vi "UpdateGraphsTableDisplay.vi"(9 "MainMenu_In":refnum<vi>, 10 "DisplayGraphsTable_In":refnum<vi>, 11 "Output Values of Device":refnum<vi>) -> ()   [LabVIEW 2013]
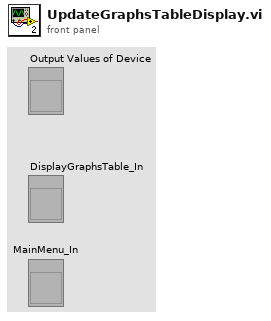
[diagram p1: front panel]
types:
  T1 = typedef "DysplayGraph.ctl" = cluster{"Graph":cluster{"X":dbl, "Y":dbl}[], "X is":u16, "Y is":u16}
  T2 = cluster{"KEITHLEY2182andKEITHLEY6221":T1, "OtherDevices":T1, "Ñombining 1 and 2 graphs ":T1}
  T3 = cluster{"KEITHLEY 2182 & KEITHLEY 6221":dbl[][], "Other Devices":dbl[][]}
  T4 = cluster{"Measurement":bool, "Save Data":bool, "LoadSetting":bool, "Save setting":bool, "Reset setting":bool, "Exit":bool}
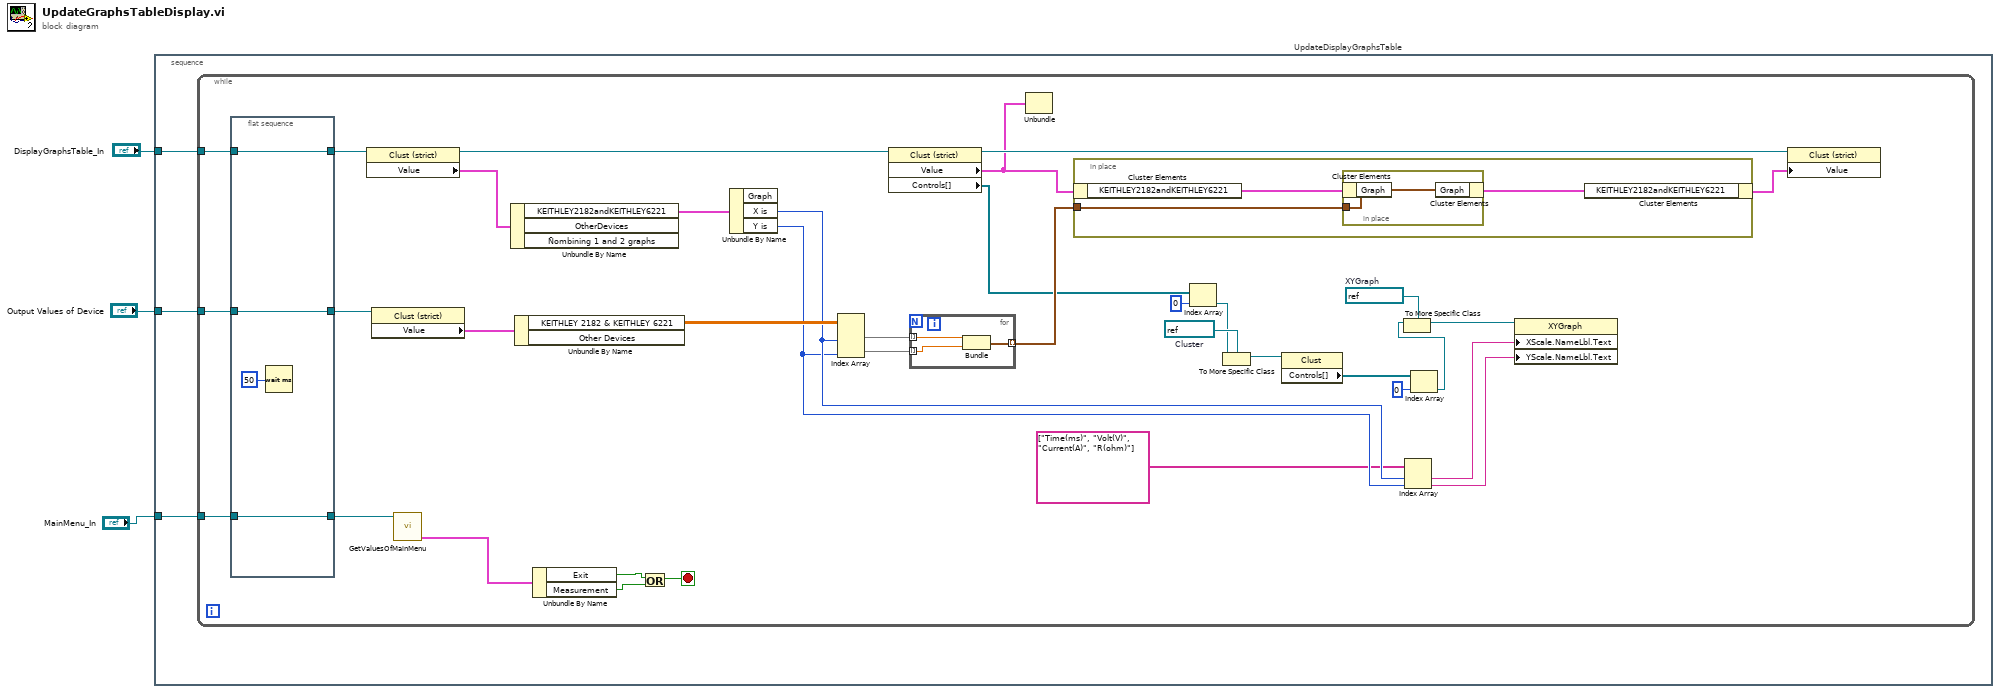
[diagram p0: block diagram]
diagram:
  n1 = stacked-sequence "UpdateDisplayGraphsTable" {
    tunnel: "DisplayGraphsTable_In" -> [w6]
    tunnel: "Output Values of Device" -> [w5]
    tunnel: "MainMenu_In" -> [w4]
    frame #0 {
      n2 = while {
        tunnel: w6 -> [w15]
        tunnel: w5 -> [w13]
        tunnel: w4 -> [w12]
        stop <- w7 stop-if-true
        w22 = refnum<vi> refnum  # Cluster
        w24 = refnum<vi> refnum  # XYGraph
        n3 = flat-sequence {
          tunnel: [w46] -> w16
          tunnel: w15 -> [w46]
          tunnel: [w45] -> w14
          tunnel: w13 -> [w45]
          tunnel: w12 -> [w44]
          tunnel: [w44] -> w11
          frame #0 {
            n4 = Wait (ms)(milliseconds to wait=u32 50) -> ()  [unwired: 1 out]
          }
        }
        n5 = property class="Clust (strict)"(reference=w16) -> (reference out=w38:refnum<vi>, "Value"=w42:T2)  [unwired: 1 in, 1 out]
        n6 = property class="Clust (strict)"(reference=w14) -> ("Value"=w37:T3)  [unwired: 1 in, 2 out]
        n7 = call "GetValuesOfMainMenu.vi"("MainMenu_In"=w11) -> ("ValuesOfMainMenu"=w17:T4)  [unwired: 9 in, 1 out]
        n8 = Unbundle By Name(w42) -> ("KEITHLEY2182andKEITHLEY6221"=w41:T1)  [unwired: 2 out]
        n9 = Unbundle By Name(w37) -> ("KEITHLEY 2182 & KEITHLEY 6221"=w36:dbl[][])  [unwired: 1 out]
        n10 = Unbundle By Name(w17) -> ("Exit"=w9:bool, "Measurement"=w8:bool)
        n11 = Or(x=w9, y=w8) -> (x .or. y?=w7:bool)
        n12 = Unbundle By Name(w41) -> ("X is"=w31:u16, "Y is"=w30:u16)  [unwired: 1 out]
        n13 = Index Array(array=w36, index (col) #1=w31, index (col) #2=w30) -> (element #1=w35:dbl[], element #2=w34:dbl[])  [unwired: 2 in]
        n14 = property class="Clust (strict)"(reference=w38) -> (reference out=w39:refnum<vi>, "Value"=w25:T2, "Controls[]"=w32:refnum<vi>[])  [unwired: 1 in, 1 out]
        n15 = for {
          tunnel: w35 -> [w49] mode=indexing
          tunnel: w34 -> [w47] mode=indexing
          tunnel: [w48] -> w33 mode=indexing
          n16 = Bundle("Numeric"=w49, "Numeric"=w47) -> (w48:cluster{"Numeric":dbl, "Numeric":dbl})  [unwired: 1 in]
        }
        n17 = Unbundle(w25) -> ()  [unwired: 3 out]
        n18 = in-place {
          in-place-border: w33 -> [w50]
          n19 = in-place-cluster #1(w25) -> ("KEITHLEY2182andKEITHLEY6221"=w52:T1)
          n20 = in-place {
            in-place-border: w50 -> [w53]
            n21 = in-place-cluster #2(w52) -> ()  [unwired: 1 out]
            n22 = in-place-cluster #2("Graph"=w53) -> (w51:T1)
          }
          n23 = in-place-cluster #1("KEITHLEY2182andKEITHLEY6221"=w51) -> (w40:T2)
        }
        n24 = Index Array(array=w32, index=0) -> (element=w21:refnum<vi>)
        n25 = To More Specific Class(target class=w22, reference=w21) -> (specific class reference=w23:refnum<vi>)  [unwired: 1 in, 1 out]
        n26 = property class="Clust"(reference=w23) -> ("Controls[]"=w19:refnum<vi>[])  [unwired: 1 in, 2 out]
        n27 = Index Array(array=string[] ["Time(ms)", "Volt(V)", "Current(A)", "R(ohm)"], index #1=w31, index #2=w30) -> (element #1=w28:string, element #2=w27:string)
        n28 = Index Array(array=w19, index=0) -> (element=w18:refnum<vi>)
        n29 = To More Specific Class(target class=w24, reference=w18) -> (specific class reference=w29:refnum<vi>)  [unwired: 1 in, 1 out]
        n30 = property class="XYGraph"(reference=w29, "XScale.NameLbl.Text"=w28, "YScale.NameLbl.Text"=w27) -> ()  [unwired: 1 in, 2 out]
        n31 = property class="Clust (strict)"(reference=w39, "Value"=w40) -> ()  [unwired: 1 in, 2 out]
      }
    }
  }
